vi "StrafeDistancePID.vi"(9 "Distance":dbl=3.0 format="%#_13g", 10 "PID gains":T1, 11 "Refnum in":refnum<k33>) -> (1 "Boolean":bool, 2 "Distance Travelled":dbl, 3 "Refnum out":refnum<k33>)   [LabVIEW 2014]
uses:
  TeleopCmd.ctl
  CmdFlag.ctl
  encoderData.vi
  <vilib>/addons/control/pid/pid.llb/PID (DBL).vi
  AutonCals.vi
  <vilib>/addons/control/pid/NI_PID_pid.lvlib
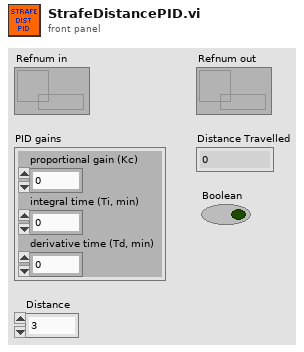
[diagram p1: front panel]
types:
  T1 = cluster{"proportional gain (Kc)":dbl, "integral time (Ti, min)":dbl, "derivative time (Td, min)":dbl}
  T2 = typedef "TeleopCmd.ctl" = cluster{"CmdFlag":T3, "throttle":dbl, "turn":dbl, "Override":bool, "Strafe":dbl, "MotorPwrMax":u8, "Time":u32, "ultrasonic override":bool}
  T3 = typedef "CmdFlag.ctl" = enum16{"noop", "logflag", "suspend", "resume"}
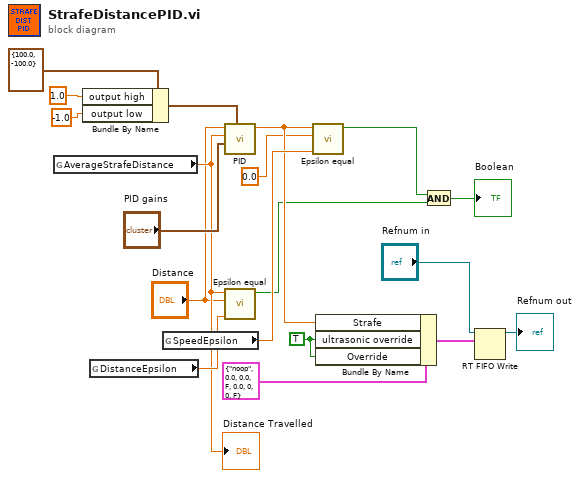
[diagram p0: block diagram]
diagram:
  w1 = TRUE ("ultrasonic override")
  n1 = global read "encoderData.vi" "AverageStrafeDistance"() -> (w15:dbl)
  "Distance Travelled" <- w15
  n2 = Bundle By Name(cluster=cluster{"output high":dbl, "output low":dbl} {"output high"=100.0, "output low"=-100.0} ("output range"), "output high"=1.0, "output low"=-1.0) -> (w3:cluster{"output high":dbl, "output low":dbl})
  n3 = global read "AutonCals.vi" "DistanceEpsilon"() -> (w16:dbl)
  n4 = global read "AutonCals.vi" "SpeedEpsilon"() -> (w17:dbl)
  n5 = call-poly <vilib>:"PID.vi"("output range"=w3, "PID gains"="PID gains", "process variable"=w15, "setpoint"="Distance") -> ("output"=w11:dbl)  [unwired: 6 in, 1 out]
  n6 = call "Epsilon equal.vi"("Epsilon"=w16, "Value2"="Distance", "Value1"=w15) -> ("Boolean"=w9:bool)  [unwired: 8 in]
  n7 = call "Epsilon equal.vi"("Epsilon"=w17, "Value2"=0.0, "Value1"=w11) -> ("Boolean"=w8:bool)  [unwired: 8 in]
  n8 = Bundle By Name(cluster=T2 {"CmdFlag"=enum."noop", "throttle"=0.0, "turn"=0.0, "Override"=FALSE, "Strafe"=0.0, "MotorPwrMax"=0, "Time"=0, "ultrasonic override"=FALSE} ("Cluster"), "Strafe"=w11, "ultrasonic override"=w1, "Override"=w1) -> (w12:T2)
  n9 = And(x=w8, y=w9) -> (x .and. y?=→"Boolean":bool)
  n10 = RT FIFO Write(0:"Refnum in", 1:w12) -> (8:→"Refnum out":refnum<k33>)  [unwired: 3 in, 3 out]
